vi "Manage RT files.vi"(7 "CONFIGURATION CLUSTER IN":T2, 8 "SAVE MODE":enum16{"DO NOT SAVE", "SAVE .CNF FILE"}(ring), 9 "PROCESSING MODE":T3(ring), 11 "R/T FILE INFORMATION IN":T4(array[cluster])) -> (1 "FILE INFO":T1(array[cluster]), 2 "R/T BREAKPOINTS":cluster{dbl, dbl}[][](array[cluster]), 3 "R/T FILE INFORMATION OUT":T4(array[cluster]), 4 "COMMENT AREA (9 FIRST ROWS)":string[][](array[string]), 5 "UNMODIFIED CONFIGURATION CLUSTER":T2)   [LabVIEW 2012]
doc: "Read, edit and save the RT information file.\nThis file contains names etc. of the \navailable resistance-to-temperature \ncalibration text files. Reads the calibration\nfiles into memory."
uses:
  <vilib>/Utility/error.llb/DialogType.ctl
panel:
  out "INFOSTRING 2":string
  in  "DISCARD":bool
  in  "ACCEPT":bool
  in  "EDIT INFO":T4(array[cluster])
  out "INFOSTRING 1":string
  # "Manage RT Files.vi"
  # "Read and edit R/T information files"
  # "Read R/T calibration files"
  # "SENSOR CHANNEL"
  # "OHMS"
  # "BREAKPOINT No."
  # "KELVINS"
  # "(Select these modes before starting\n  the VI)"
  # "SENSOR CHANNEL"
  # "(ROW)"
  # "SENSOR. CHANNEL"
  # "FILE READ INFO"
  # "AND PROCEED"
  # "This VI has four processing modes and two file save modes. The modes must be selected before starting the VI:\n1) NONE:  The RT  input cluster is passed transparently through the VI.  depending on the file save mode, it can be saved or not saved.\n2) READ: The VI tries to read \"avs47B_rt_file_info.cnf\" from the operating directory. If success, the file is read and returned as the output RT cluster. If failed, a default cluster is returned as output. It can be saved or not saved.\n3) READ AND EDIT: The VI tries to open  \"avs47B_rt_file_info.cnf\" from the operating directory. If success, the file contents is presented for editing. You can edit the settings of various input channels by selecting the channel and then selecting the required settings. The names of the RT calibration files have to be typed, other parameters can be only selected. After editing, select either \"accept edits\" or \"discard edits\" and the VI proceeds to next section, where the RT information can be saved or not saved.\n4) DEFAULTS: Default RT information is unconditionally returned as output. It can be saved or not saved."
  # "INPUT CHANNEL"
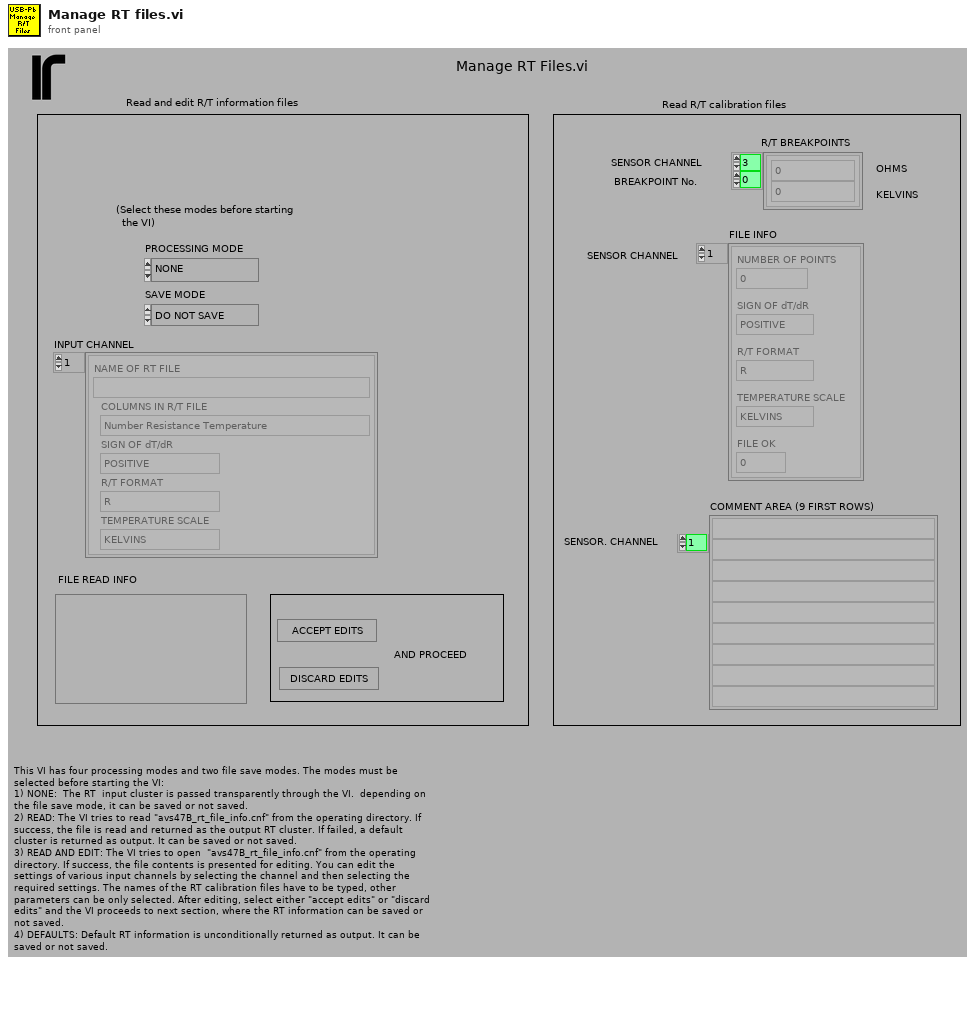
[diagram p1: front panel]
types:
  T1 = cluster{"NUMBER OF POINTS":i32, "SIGN OF dT/dR":enum16{"POSITIVE", "NEGATIVE"}, "R/T FORMAT ":enum16{"R", "LOG(R)"}, "TEMPERATURE SCALE":enum16{"KELVINS", "CELSIUS"}, "FILE OK":i32}[]
  T2 = cluster{"VISA RESOURCE":refnum<visa-resource-name>, "PICOBUS ADDRESS":u8, "DISABLE AL":u8, "REMOTE":u8, "INPUT":u8, "CHANNEL":u8, "RANGE":u8, "EXCITATION":u8, "DISPLAY":u8, "DIGITAL REFERENCE":u16, "SET POINT":dbl, "PROP GAIN":u8, "INTG":u8, "DERIV":u8, "POWER BIAS":u8, "POWER RANGE":u8, "INFO STRING":string, "HEATER RESISTANCE":dbl, "INTERVAL":u8, " SENSOR dR/dT":u8}
  T3 = enum16{"NONE", "READ", "READ AND EDIT", "DEFAULTS"}
  T4 = cluster{"NAME OF RT FILE":string, "COLUMNS IN R/T FILE":enum16{"Number Resistance Temperature", "Resistance Temperature"}, "SIGN OF dT/dR":enum16{"POSITIVE", "NEGATIVE"}, "R/T FORMAT ":enum16{"R", "LOG(R)"}, "TEMPERATURE SCALE":enum16{"KELVINS", "CELSIUS"}}[]
  T5 = enum16{"Number Resistance Temperature", "Resistance Temperature"}
  T6 = cluster{"NAME OF RT FILE":string, "COLUMNS IN R/T FILE":enum16{"Number Resistance Temperature", "Resistance Temperature"}, "SIGN OF dT/dR":enum16{"POSITIVE", "NEGATIVE"}, "R/T FORMAT ":enum16{"R", "LOG(R)"}, "TEMPERATURE SCALE":enum16{"KELVINS", "CELSIUS"}}
  T7 = enum16{"open", "replace", "create", "open or create", "replace or create", "replace or create with confirmation"}
  T8 = typedef "DialogType.ctl" = u16
  T9 = cluster{"NUMBER OF POINTS":i32, "SIGN OF dT/dR":enum16{"POSITIVE", "NEGATIVE"}, "R/T FORMAT ":enum16{"R", "LOG(R)"}, "TEMPERATURE SCALE":enum16{"KELVINS", "CELSIUS"}, "FILE OK":i32}
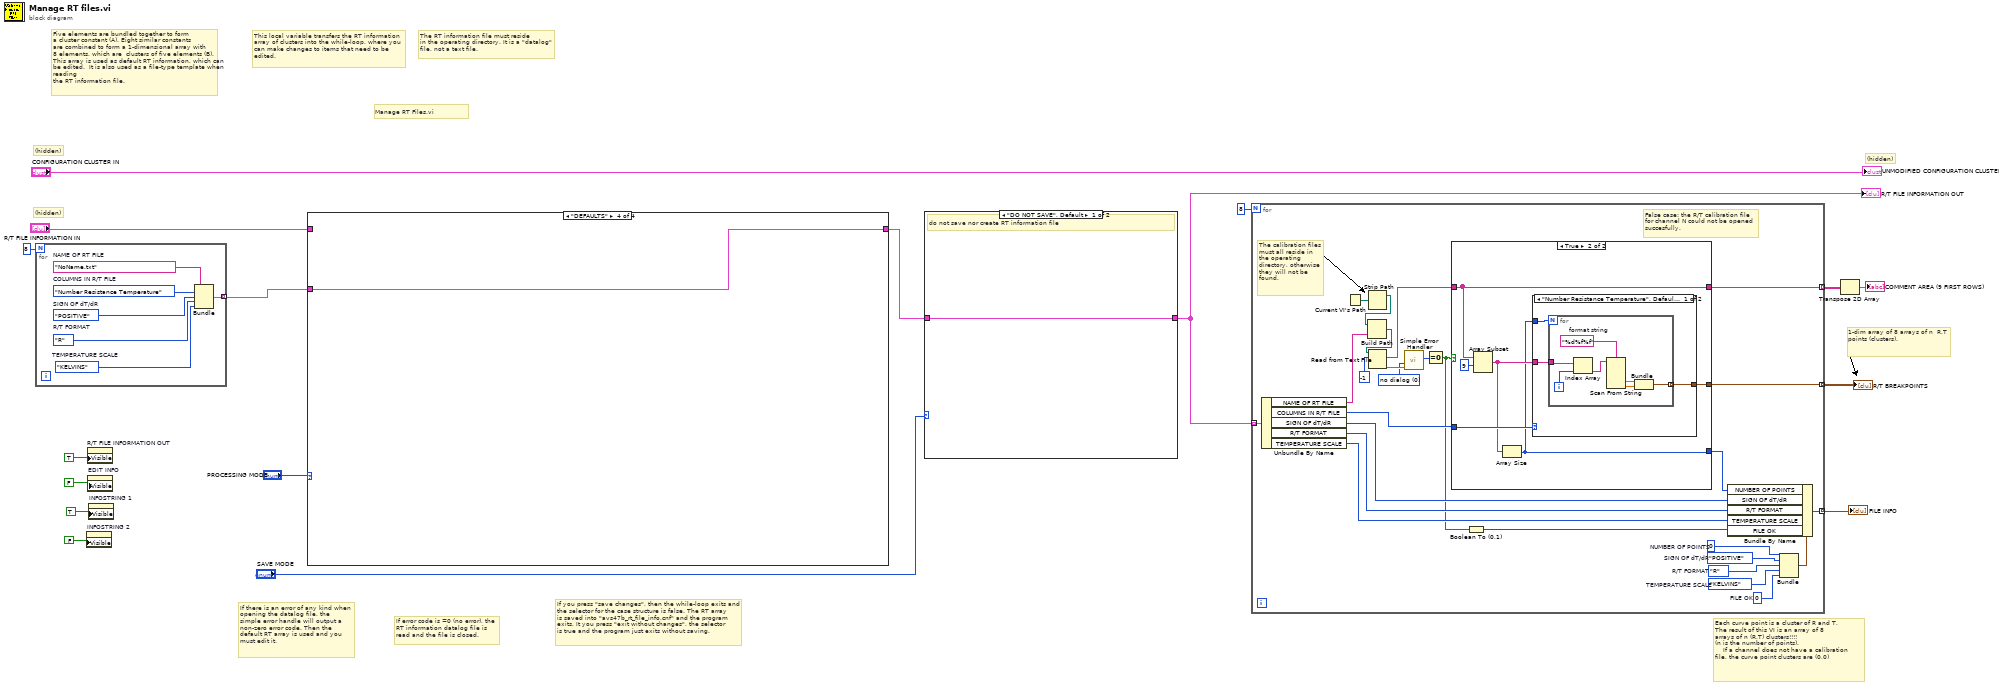
[diagram p0: block diagram]
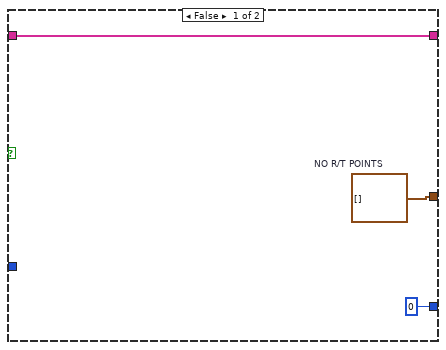
[diagram p2: hidden frame]
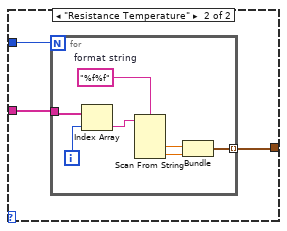
[diagram p3: hidden frame]
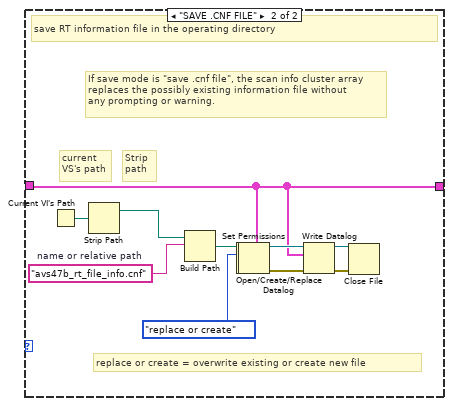
[diagram p4: hidden frame]
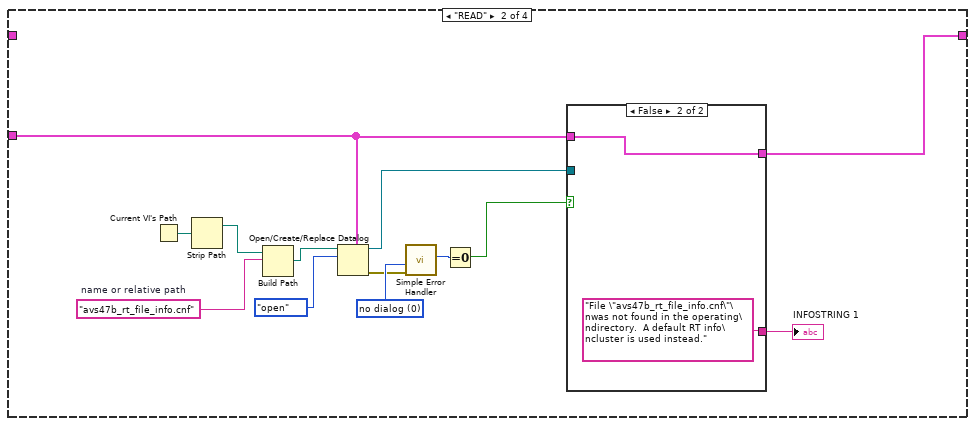
[diagram p6: hidden frame]
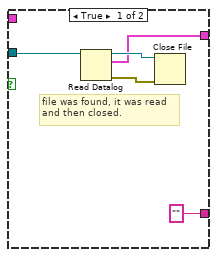
[diagram p7: hidden frame]
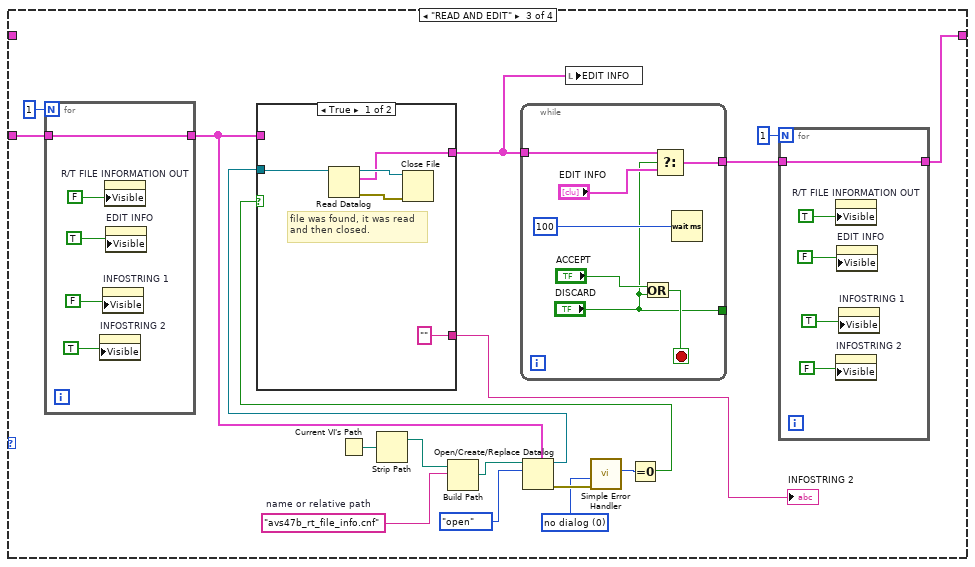
[diagram p8: hidden frame]
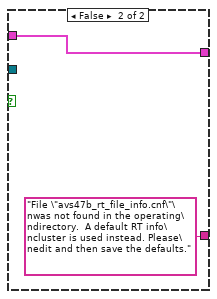
[diagram p9: hidden frame]
diagram:
  # "(hidden)"
  # "(hidden)"
  # "1-dim array of 8 arrays of n  R,T points (clusters)."
  # "Each curve point is a cluster of R and T,\nThe result of this VI is an array of 8 \narrays of n (R,T) clusters!!!!\n(n is the number of points).\n    If a channel does not have a calibration\nfile, the curve point clusters are (0,0)"
  # "(hidden)"
  # "If you press \"save changes\", then the while-loop exits and\nthe selector for the case structure is false. The RT array\nis saved into \"avs47b_rt_file_info.cnf\" and the program\nexits. It you press \"exit without changes\", the selector \nis true and the program just exits without saving."
  # "This local variable transfers the RT information\narray of clusters into the while-loop, where you\ncan make changes to items that need to be \nedited."
  # "If error code is =0 (no error), the\nRT information datalog file is \nread and the file is closed."
  # "If there is an error of any kind when\nopening the datalog file, the \nsimple error handle will output a\nnon-zero error code. Then the\ndefault RT array is used and you\nmust edit it."
  # "The RT information file must reside\nin the operating directory. It is a \"datalog\"\nfile, not a text file."
  # "Five elements are bundled together to form\na cluster constant (A). Eight similar constants\nare combined to form a 1-dimensional array with\n8 elements, which are  clusters of five elements (B). This array is used as default RT information, which can be edited.  It is also used as a file-type template when reading\nthe RT information file."
  # "Manage RT Files.vi"
  n1 = for {
    N: 8 -> [_]
    tunnel: [w19] -> w16 mode=indexing
    w18 = enum16{"KELVINS", "CELSIUS"}."KELVINS"  # TEMPERATURE SCALE
    w20 = enum16{"R", "LOG(R)"}."R"  # R/T FORMAT
    w21 = enum16{"POSITIVE", "NEGATIVE"}."POSITIVE"  # SIGN OF dT/dR
    w22 = T5."Number Resistance Temperature"  # COLUMNS IN R/T FILE
    w23 = "NoName.txt"  # NAME OF RT FILE
    n2 = Bundle("NAME OF RT FILE"=w23, "COLUMNS IN R/T FILE"=w22, "SIGN OF dT/dR"=w21, "R/T FORMAT"=w20, "TEMPERATURE SCALE"=w18) -> (w19:T6)  [unwired: 1 in]
  }
  n3 = property on="INFOSTRING 2" class="Str"("Visible"=FALSE) -> ()  [unwired: 2 in, 2 out]
  n4 = property on="R/T FILE INFORMATION OUT" class="Arr (strict)"("Visible"=TRUE) -> ()  [unwired: 2 in, 2 out]
  n5 = property on="EDIT INFO" class="Arr (strict)"("Visible"=FALSE) -> ()  [unwired: 2 in, 2 out]
  n6 = property on="INFOSTRING 1" class="Str"("Visible"=TRUE) -> ()  [unwired: 2 in, 2 out]
  n7 = case shown="\"DEFAULTS\"" "PROCESSING MODE" {
    tunnel: w16 -> [_ w27 w51 w87]
    tunnel: "R/T FILE INFORMATION IN" -> [w24 _ _ _]
    tunnel: [w24 w26 w46 w87] -> w11
    frame "NONE", Default {
    }
    frame "READ" {
      w32 = T8 0 items=["no dialog", "OK message", "continue or stop message", "OK message + warnings", "continue/stop + warnings"] ("type of dialog (OK msg:1)")
      w28 = "avs47b_rt_file_info.cnf"  # name or relative path
      n8 = Current VI's Path() -> (path=w29:path)
      n9 = Strip Path(path=w29) -> (stripped path=w30:path)  [unwired: 1 out]
      n10 = Build Path(base path=w30, name or relative path=w28) -> (appended path=w36:path)
      n11 = Open/Create/Replace Datalog(5:w27, 10:T7."open" ("operation (0:open)"), 11:w36) -> (0:w31:errorcluster, 3:w37:refnum<k1>)  [unwired: 3 in, 1 out]
      n12 = call <vilib>:"Simple Error Handler.vi"("type of dialog (OK msg:1)"=w32, "error in (no error)"=w31) -> ("code out"=w34:i32)  [unwired: 3 in, 4 out]
      n13 = Equal To 0?(x=w34) -> (x = 0?=w35:bool)
      n14 = case shown="False" w35 {
        tunnel: w37 -> [w38 _]
        tunnel: w27 -> [_ w44]
        tunnel: [w40 w44] -> w26
        tunnel: ["" "File \"avs47b_rt_file_info.cnf\"\nwas not found in the operating\ndirectory.  A default RT info\ncluster is used instead."] -> w25
        frame True {
          # "file was found, it was read\nand then closed."
          n15 = Read Datalog(7:w38) -> (0:w42:errorcluster, 2:w40:T4, 3:w41:refnum<k1>)  [unwired: 2 in]
          n16 = Close File(refnum=w41, error in=w42) -> ()  [unwired: 2 out]
        }
        frame False {
        }
      }
      "INFOSTRING 1" <- w25
    }
    frame "READ AND EDIT" {
      w58 = T8 0 items=["no dialog", "OK message", "continue or stop message", "OK message + warnings", "continue/stop + warnings"] ("type of dialog (OK msg:1)")
      w62 = "avs47b_rt_file_info.cnf"  # name or relative path
      n17 = for {
        N: 1 -> [_]
        tunnel: w51 -> [w72]
        tunnel: [w72] -> w50
        n18 = property on="INFOSTRING 2" class="Str"("Visible"=TRUE) -> ()  [unwired: 2 in, 2 out]
        n19 = property on="INFOSTRING 1" class="Str"("Visible"=FALSE) -> ()  [unwired: 2 in, 2 out]
        n20 = property on="R/T FILE INFORMATION OUT" class="Arr (strict)"("Visible"=FALSE) -> ()  [unwired: 2 in, 2 out]
        n21 = property on="EDIT INFO" class="Arr (strict)"("Visible"=TRUE) -> ()  [unwired: 2 in, 2 out]
      }
      n22 = Current VI's Path() -> (path=w61:path)
      n23 = Strip Path(path=w61) -> (stripped path=w60:path)  [unwired: 1 out]
      n24 = Build Path(base path=w60, name or relative path=w62) -> (appended path=w53:path)
      n25 = Open/Create/Replace Datalog(5:w50, 10:T7."open" ("operation (0:open)"), 11:w53) -> (0:w59:errorcluster, 3:w52:refnum<k1>)  [unwired: 3 in, 1 out]
      n26 = call <vilib>:"Simple Error Handler.vi"("type of dialog (OK msg:1)"=w58, "error in (no error)"=w59) -> ("code out"=w56:i32)  [unwired: 3 in, 4 out]
      n27 = Equal To 0?(x=w56) -> (x = 0?=w54:bool)
      n28 = case shown="True" w54 {
        tunnel: w52 -> [w80 _]
        tunnel: w50 -> [_ w86]
        tunnel: [w82 w86] -> w55
        tunnel: ["" "File \"avs47b_rt_file_info.cnf\"\nwas not found in the operating\ndirectory.  A default RT info\ncluster is used instead. Please\nedit and then save the defaults."] -> w45
        frame True {
          # "file was found, it was read\nand then closed."
          n29 = Read Datalog(7:w80) -> (0:w84:errorcluster, 2:w82:T4, 3:w83:refnum<k1>)  [unwired: 2 in]
          n30 = Close File(refnum=w83, error in=w84) -> ()  [unwired: 2 out]
        }
        frame False {
        }
      }
      "INFOSTRING 2" <- w45
      n31 = while {
        tunnel: w55 -> [w76]
        tunnel: ["DISCARD"] -> _
        tunnel: [w74] -> w47
        stop <- w78 stop-if-true
        n32 = Or(x="ACCEPT", y="DISCARD") -> (x .or. y?=w78:bool)
        n33 = Select(t=w76, s="DISCARD", f="EDIT INFO") -> (s? t:f=w74:T4)
        n34 = Wait (ms)(milliseconds to wait=u32 100) -> ()  [unwired: 1 out]
      }
      n35 = local write "EDIT INFO"(w55) -> ()
      n36 = for {
        N: 1 -> [_]
        tunnel: w47 -> [w67]
        tunnel: [w67] -> w46
        n37 = property on="R/T FILE INFORMATION OUT" class="Arr (strict)"("Visible"=TRUE) -> ()  [unwired: 2 in, 2 out]
        n38 = property on="INFOSTRING 2" class="Str"("Visible"=FALSE) -> ()  [unwired: 2 in, 2 out]
        n39 = property on="EDIT INFO" class="Arr (strict)"("Visible"=FALSE) -> ()  [unwired: 2 in, 2 out]
        n40 = property on="INFOSTRING 1" class="Str"("Visible"=TRUE) -> ()  [unwired: 2 in, 2 out]
      }
    }
    frame "DEFAULTS" {
    }
  }
  n41 = case shown="\"DO NOT SAVE\", Default" "SAVE MODE" {
    tunnel: [w88 w89] -> w4
    tunnel: w11 -> [w88 w89]
    frame "DO NOT SAVE", Default {
      # "do not save nor create RT information file"
    }
    frame "SAVE .CNF FILE" {
      w94 = "avs47b_rt_file_info.cnf"  # name or relative path
      # "If save mode is \"save .cnf file\", the scan info cluster array\nreplaces the possibly existing information file without \nany prompting or warning."
      # "Strip\npath"
      # "current\nVS's path"
      # "replace or create = overwrite existing or create new file"
      # "save RT information file in the operating directory"
      n42 = Current VI's Path() -> (path=w96:path)
      n43 = Strip Path(path=w96) -> (stripped path=w97:path)  [unwired: 1 out]
      n44 = Build Path(base path=w97, name or relative path=w94) -> (appended path=w95:path)
      n45 = Open/Create/Replace Datalog(5:w89, 10:T7."replace or create" ("operation (0:open)"), 11:w95) -> (0:w98:errorcluster, 3:w90:refnum<k1>)  [unwired: 3 in, 1 out]
      n46 = Set Permissions(8:w98, 11:w95) -> (0:w91:errorcluster)  [unwired: 3 in, 1 out]
      n47 = Write Datalog(4:w91, 6:w89, 7:w90) -> (0:w93:errorcluster, 3:w92:refnum<k1>)
      n48 = Close File(refnum=w92, error in=w93) -> ()  [unwired: 2 out]
    }
  }
  "R/T FILE INFORMATION OUT" <- w4
  n49 = for {
    N: 8 -> [_]
    tunnel: [w117] -> w3 mode=indexing
    tunnel: w4 -> [w116] mode=indexing
    tunnel: [w113] -> w5 mode=indexing
    tunnel: [w106] -> w2 mode=indexing
    w101 = 0  # FILE OK
    w104 = enum16{"KELVINS", "CELSIUS"}."KELVINS"  # TEMPERATURE SCALE
    w105 = enum16{"R", "LOG(R)"}."R"  # R/T FORMAT
    w109 = enum16{"POSITIVE", "NEGATIVE"}."POSITIVE"  # SIGN OF dT/dR
    w110 = 0  # NUMBER OF POINTS
    w120 = T8 0 items=["no dialog", "OK message", "continue or stop message", "OK message + warnings", "continue/stop + warnings"] ("type of dialog (OK msg:1)")
    # "False case: the R/T calibration file\nfor channel N could not be opened\nsuccesfully."
    # "The calibration files\nmust all reside in\nthe operating\ndirectory, otherwise\nthey will not be\nfound."
    n50 = Unbundle By Name(w116) -> ("NAME OF RT FILE"=w115:string, "COLUMNS IN R/T FILE"=w114:T5, "SIGN OF dT/dR"=w108:enum16{"POSITIVE", "NEGATIVE"}, "R/T FORMAT"=w107:enum16{"R", "LOG(R)"}, "TEMPERATURE SCALE"=w103:enum16{"KELVINS", "CELSIUS"})
    n51 = Current VI's Path() -> (path=w124:path)
    n52 = Strip Path(path=w124) -> (stripped path=w125:path)  [unwired: 1 out]
    n53 = Build Path(base path=w125, name or relative path=w115) -> (appended path=w123:path)
    n54 = Read from Text File(file (use dialog)=w123, count=-1) -> (text=w118:string[], error out=w121:errorcluster)  [unwired: 2 in, 2 out]
    n55 = call <vilib>:"Simple Error Handler.vi"("type of dialog (OK msg:1)"=w120, "error in (no error)"=w121) -> ("code out"=w119:i32)  [unwired: 3 in, 4 out]
    n56 = Equal To 0?(x=w119) -> (x = 0?=w102:bool)
    n57 = case shown="True" w102 {
      tunnel: [w127 w133] -> w117
      tunnel: w114 -> [_ w132]
      tunnel: w118 -> [w126 w130]
      tunnel: [0 w129] -> w111
      tunnel: [w126 w130] -> w113
      frame False {
        w127 = cluster{dbl, dbl}[] []  # NO R/T POINTS
      }
      frame True {
        n58 = Array Subset(array=w130, index=9) -> (w131:string[])  [unwired: 1 in]
        n59 = Array Size(array=w131) -> (size(s)=w129:i32)
        n60 = case shown="\"Number Resistance Temperature\", Default" w132 {
          tunnel: w131 -> [w137 w146]
          tunnel: [w136 w147] -> w133
          tunnel: w129 -> [w135 w145]
          frame "Number Resistance Temperature", Default {
            n61 = for {
              N: w135 -> [_]
              tunnel: w137 -> [w144]
              tunnel: [w138] -> w136 mode=indexing
              i -> [w143]
              w141 = "%d%f%f"  # format string
              n62 = Index Array(array=w144, index=w143) -> (element=w142:string)
              n63 = Scan From String(format string=w141, input string=w142) -> (output 2=w140:dbl, output 3=w139:dbl)  [unwired: 6 in, 3 out]
              n64 = Bundle(w140, w139) -> (w138:cluster{dbl, dbl})  [unwired: 1 in]
            }
          }
          frame "Resistance Temperature" {
            n65 = for {
              N: w145 -> [_]
              tunnel: w146 -> [w154]
              tunnel: [w150] -> w147 mode=indexing
              i -> [w153]
              w151 = "%f%f"  # format string
              n66 = Index Array(array=w154, index=w153) -> (element=w152:string)
              n67 = Scan From String(format string=w151, input string=w152) -> (output 1=w149:dbl, output 2=w148:dbl)  [unwired: 4 in, 3 out]
              n68 = Bundle(w149, w148) -> (w150:cluster{dbl, dbl})  [unwired: 1 in]
            }
          }
        }
      }
    }
    n69 = Boolean To (0,1)(Boolean=w102) -> (0, 1=w100:i16)
    n70 = Bundle("NUMBER OF POINTS"=w110, "SIGN OF dT/dR"=w109, "R/T FORMAT"=w105, "TEMPERATURE SCALE"=w104, "FILE OK"=w101) -> (w112:T9)  [unwired: 1 in]
    n71 = Bundle By Name(cluster=w112, "NUMBER OF POINTS"=w111, "SIGN OF dT/dR"=w108, "R/T FORMAT"=w107, "TEMPERATURE SCALE"=w103, "FILE OK"=w100) -> (w106:T9)
  }
  "R/T BREAKPOINTS" <- w3
  "FILE INFO" <- w2
  n72 = Transpose 2D Array(2D array=w5) -> (transposed array=→"COMMENT AREA (9 FIRST ROWS)":string[][])
  "UNMODIFIED CONFIGURATION CLUSTER" <- "CONFIGURATION CLUSTER IN"
